vi "messages.vi"() -> ()   [LabVIEW 2017]
uses:
  C:/Users/LukashPC/Desktop/projekt_paczkomat/projekt_paczkomat/wiadomosci.ctl
  C:/Users/LukashPC/Desktop/projekt_paczkomat/projekt_paczkomat/komunikaty_przy_przyciskach.ctl
panel:
  out "Message":string
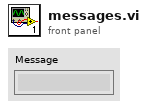
[diagram p1: front panel]
types:
  T1 = typedef "komunikaty_przy_przyciskach.ctl" = string[][]
  T2 = typedef "wiadomosci.ctl" = string[][]
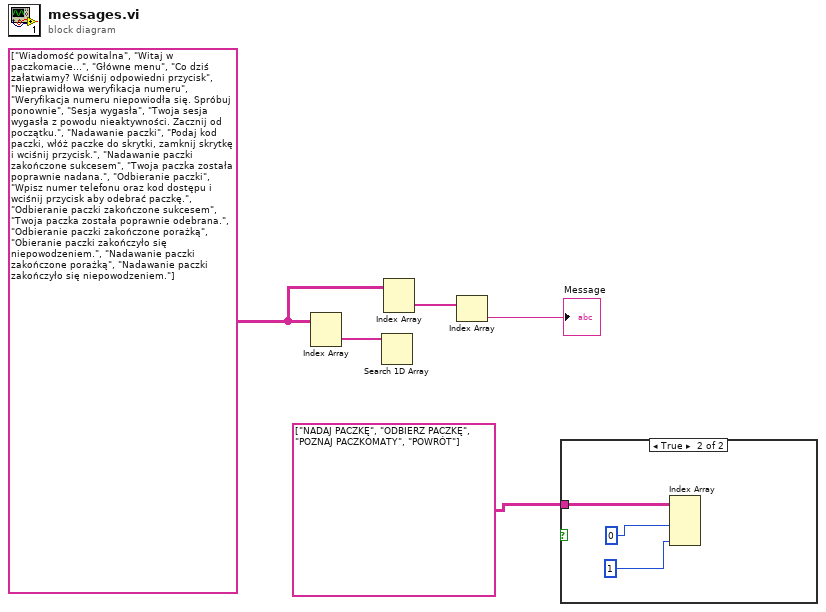
[diagram p0: block diagram]
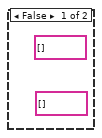
[diagram p2: hidden frame]
diagram:
  w4 = T2 [["Wiadomość powitalna", "Witaj w paczkomacie..."], ["Główne menu", "Co dziś załatwiamy? Wciśnij odpowiedni przycisk"], ["Nieprawidłowa weryfikacja numeru", "Weryfikacja numeru niepowiodła się. Spróbuj ponownie"], ["Sesja wygasła", "Twoja sesja wygasła z powodu nieaktywności. Zacznij od początku."], ["Nadawanie paczki", "Podaj kod paczki, włóż paczke do skrytki, zamknij skrytkę i wciśnij przycisk."], ["Nadawanie paczki zakończone sukcesem", "Twoja paczka została poprawnie nadana."], ["Odbieranie paczki", "Wpisz numer telefonu oraz kod dostępu i wciśnij przycisk aby odebrać paczkę."], ["Odbieranie paczki zakończone sukcesem", "Twoja paczka została poprawnie odebrana."], ["Odbieranie paczki zakończone porażką", "Obieranie paczki zakończyło się niepowodzeniem."], ["Nadawanie paczki zakończone porażką", "Nadawanie paczki zakończyło się niepowodzeniem."]] ("Array")
  n1 = Index Array(array=w4) -> (element=w5:string[])  [unwired: 2 in]
  n2 = Search 1D Array(1D array=w5) -> ()  [unwired: 2 in, 1 out]
  n3 = Index Array(array=w4) -> (element=w3:string[])  [unwired: 2 in]
  n4 = Index Array(array=w3) -> (element=→"Message":string)  [unwired: 1 in]
  n5 = case shown="\"Menu\"" {
    selector: _ -> [_ _]
    tunnel: T1 [["NADAJ PACZKĘ", "ODBIERZ PACZKĘ"], ["POZNAJ PACZKOMATY", "POWRÓT"]] ("Array") -> [_ w8]
    frame False {
      (unwired) string[] []
      (unwired) string[] []
    }
    frame True {
      n6 = Index Array(array=w8, index (col) #1=0, index (col) #2=1) -> ()  [unwired: 2 in, 2 out]
    }
  }
